vi "PRBS64 Parallel Tx - N Lanes.vi"(6 "ready for output (T)":bool=TRUE, 7 "reset":bool, 11 "seed":u64[](array[numeric])) -> (1 "output valid":bool, 3 "sequence out":u64[](array[numeric]))   [LabVIEW 2023, in "Aurora64b66b Utilities FPGA.lvlib"]
uses:
  Aurora64b66b Utilities FPGA.lvlib
  Program Files/NI/LVAddons/niidl/1/instr.lib/_niInstr/Basic Elements/v1/FPGA/niInstr Basic Elements v1 FPGA.lvlib
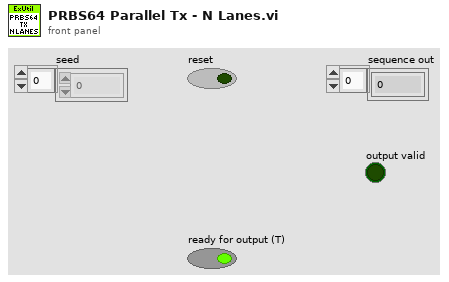
[diagram p1: front panel]
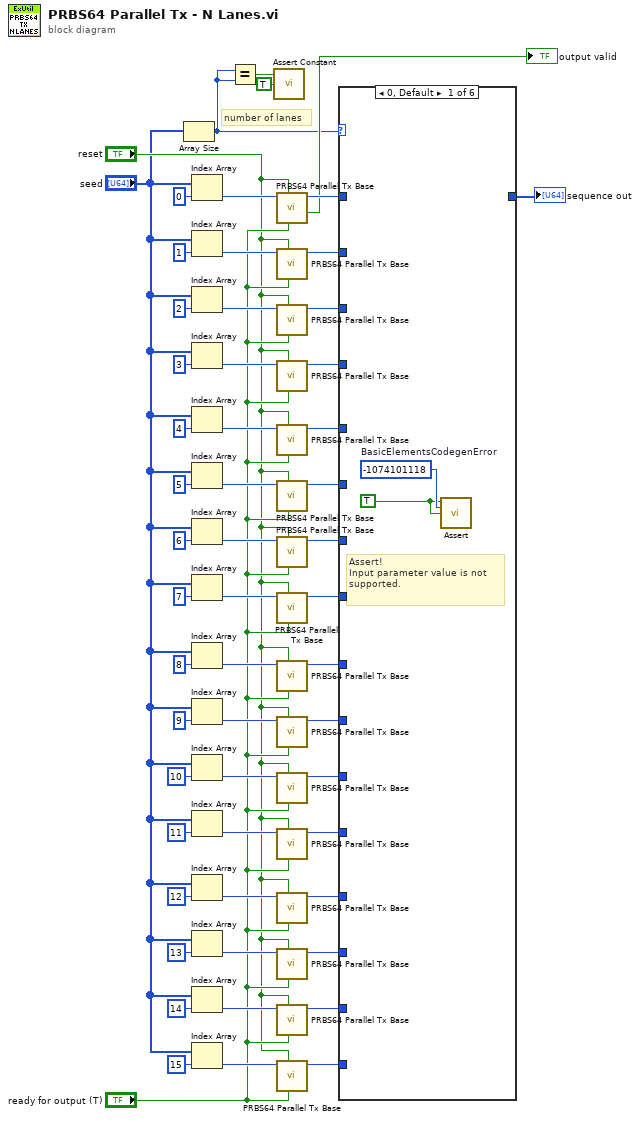
[diagram p0: block diagram]
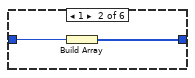
[diagram p2: hidden frame]
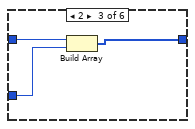
[diagram p3: hidden frame]
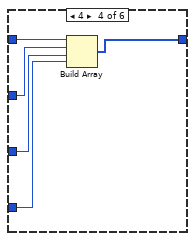
[diagram p4: hidden frame]
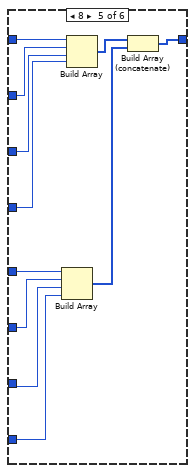
[diagram p5: hidden frame]
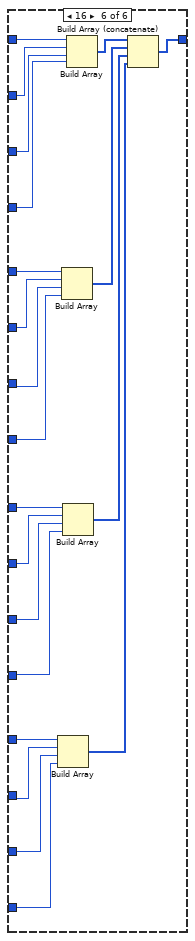
[diagram p6: hidden frame]
diagram:
  # "number of lanes"
  n1 = Array Size(array="seed") -> (size(s)=w1:i32)
  n2 = Index Array(array="seed", index=0) -> (element=w55:u64)
  n3 = Index Array(array="seed", index=1) -> (element=w51:u64)
  n4 = Index Array(array="seed", index=2) -> (element=w50:u64)
  n5 = Index Array(array="seed", index=3) -> (element=w49:u64)
  n6 = Index Array(array="seed", index=4) -> (element=w38:u64)
  n7 = Index Array(array="seed", index=5) -> (element=w42:u64)
  n8 = Index Array(array="seed", index=6) -> (element=w43:u64)
  n9 = Index Array(array="seed", index=7) -> (element=w44:u64)
  n10 = Index Array(array="seed", index=8) -> (element=w31:u64)
  n11 = Index Array(array="seed", index=9) -> (element=w27:u64)
  n12 = Index Array(array="seed", index=10) -> (element=w26:u64)
  n13 = Index Array(array="seed", index=11) -> (element=w25:u64)
  n14 = Index Array(array="seed", index=12) -> (element=w18:u64)
  n15 = Index Array(array="seed", index=13) -> (element=w22:u64)
  n16 = Index Array(array="seed", index=14) -> (element=w23:u64)
  n17 = Index Array(array="seed", index=15) -> (element=w24:u64)
  n18 = Equal?(x=w1, y=w1) -> (x = y?=w3:bool)
  n19 = call "Assert Constant.vi"("constant terminal"=w3, "enable show error"=TRUE) -> ()  [unwired: 14 in]
  n20 = call "PRBS64 Parallel Tx Base.vi"("ready for output (T)"="ready for output (T)", "reset"="reset", "seed"=w55) -> ("output valid"=→"output valid":bool, "prbs tx"=w48:u64)  [unwired: 7 in]
  n21 = call "PRBS64 Parallel Tx Base.vi"("ready for output (T)"="ready for output (T)", "reset"="reset", "seed"=w51) -> ("prbs tx"=w47:u64)  [unwired: 7 in, 1 out]
  n22 = call "PRBS64 Parallel Tx Base.vi"("ready for output (T)"="ready for output (T)", "reset"="reset", "seed"=w50) -> ("prbs tx"=w46:u64)  [unwired: 7 in, 1 out]
  n23 = call "PRBS64 Parallel Tx Base.vi"("ready for output (T)"="ready for output (T)", "reset"="reset", "seed"=w49) -> ("prbs tx"=w45:u64)  [unwired: 7 in, 1 out]
  n24 = call "PRBS64 Parallel Tx Base.vi"("ready for output (T)"="ready for output (T)", "reset"="reset", "seed"=w38) -> ("prbs tx"=w36:u64)  [unwired: 7 in, 1 out]
  n25 = call "PRBS64 Parallel Tx Base.vi"("ready for output (T)"="ready for output (T)", "reset"="reset", "seed"=w42) -> ("prbs tx"=w35:u64)  [unwired: 7 in, 1 out]
  n26 = call "PRBS64 Parallel Tx Base.vi"("ready for output (T)"="ready for output (T)", "reset"="reset", "seed"=w43) -> ("prbs tx"=w34:u64)  [unwired: 7 in, 1 out]
  n27 = call "PRBS64 Parallel Tx Base.vi"("ready for output (T)"="ready for output (T)", "reset"="reset", "seed"=w44) -> ("prbs tx"=w33:u64)  [unwired: 7 in, 1 out]
  n28 = call "PRBS64 Parallel Tx Base.vi"("ready for output (T)"="ready for output (T)", "reset"="reset", "seed"=w31) -> ("prbs tx"=w14:u64)  [unwired: 7 in, 1 out]
  n29 = call "PRBS64 Parallel Tx Base.vi"("ready for output (T)"="ready for output (T)", "reset"="reset", "seed"=w27) -> ("prbs tx"=w13:u64)  [unwired: 7 in, 1 out]
  n30 = call "PRBS64 Parallel Tx Base.vi"("ready for output (T)"="ready for output (T)", "reset"="reset", "seed"=w26) -> ("prbs tx"=w12:u64)  [unwired: 7 in, 1 out]
  n31 = call "PRBS64 Parallel Tx Base.vi"("ready for output (T)"="ready for output (T)", "reset"="reset", "seed"=w25) -> ("prbs tx"=w11:u64)  [unwired: 7 in, 1 out]
  n32 = call "PRBS64 Parallel Tx Base.vi"("ready for output (T)"="ready for output (T)", "reset"="reset", "seed"=w18) -> ("prbs tx"=w10:u64)  [unwired: 7 in, 1 out]
  n33 = call "PRBS64 Parallel Tx Base.vi"("ready for output (T)"="ready for output (T)", "reset"="reset", "seed"=w22) -> ("prbs tx"=w9:u64)  [unwired: 7 in, 1 out]
  n34 = call "PRBS64 Parallel Tx Base.vi"("ready for output (T)"="ready for output (T)", "reset"="reset", "seed"=w23) -> ("prbs tx"=w8:u64)  [unwired: 7 in, 1 out]
  n35 = call "PRBS64 Parallel Tx Base.vi"("ready for output (T)"="ready for output (T)", "reset"="reset", "seed"=w24) -> ("prbs tx"=w7:u64)  [unwired: 7 in, 1 out]
  n36 = case shown="0, Default" w1 {
    tunnel: w48 -> [_ w60 w63 w68 w79 w100]
    tunnel: w47 -> [_ _ w61 w66 w77 w98]
    tunnel: w46 -> [_ _ _ w65 w76 w97]
    tunnel: w45 -> [_ _ _ w64 w75 w96]
    tunnel: w36 -> [_ _ _ _ w74 w95]
    tunnel: w35 -> [_ _ _ _ w73 w94]
    tunnel: w34 -> [_ _ _ _ w72 w93]
    tunnel: w33 -> [_ _ _ _ w71 w92]
    tunnel: w14 -> [_ _ _ _ _ w89]
    tunnel: w13 -> [_ _ _ _ _ w88]
    tunnel: w12 -> [_ _ _ _ _ w87]
    tunnel: w11 -> [_ _ _ _ _ w86]
    tunnel: w10 -> [_ _ _ _ _ w85]
    tunnel: w9 -> [_ _ _ _ _ w84]
    tunnel: w8 -> [_ _ _ _ _ w83]
    tunnel: w7 -> [_ _ _ _ _ w82]
    tunnel: [_ w59 w62 w67 w70 w91] -> w5
    frame 0, Default {
      w58 = -1074101118  # BasicElementsCodegenError
      w57 = TRUE ("assert")
      # "Assert!\nInput parameter value is not supported."
      n37 = call "Assert.vi"("assert"=w57, "error code"=w58, "enable show error"=w57) -> ()  [unwired: 13 in]
    }
    frame 1 {
      n38 = Build Array(w60) -> (w59:u64[])
    }
    frame 2 {
      n39 = Build Array(w63, w61) -> (w62:u64[])
    }
    frame 4 {
      n40 = Build Array(w68, w66, w65, w64) -> (w67:u64[])
    }
    frame 8 {
      n41 = Build Array(w74, w73, w72, w71) -> (w69:u64[])
      n42 = Build Array(w79, w77, w76, w75) -> (w78:u64[])
      n43 = Build Array (concatenate)(w78, w69) -> (w70:u64[])
    }
    frame 16 {
      n44 = Build Array(w85, w84, w83, w82) -> (w80:u64[])
      n45 = Build Array(w95, w94, w93, w92) -> (w90:u64[])
      n46 = Build Array(w89, w88, w87, w86) -> (w81:u64[])
      n47 = Build Array(w100, w98, w97, w96) -> (w99:u64[])
      n48 = Build Array (concatenate)(w99, w90, w81, w80) -> (w91:u64[])
    }
  }
  "sequence out" <- w5
